vi "Select DB data.vi"(6 "index":i32, 8 "error in (no error)":errorcluster caption="错误输入（无错误）", 9 "Code":string, 10 "Tabe":string, 11 "Connncet State":T1) -> (0 "error out":errorcluster caption="错误输出", 1 "data":string[][](array[string]), 2 "state":bool, 3 "Connect State":T1, 4 "data var":variant[][](array[variant]))   [LabVIEW 2014]
uses:
  <vilib>/addons/database/_DB Variant To Data/Database Variant To Data.xnode
  Ctr/Constr.ctl
  <vilib>/addons/database/Connection.llb/Conn ObjectReference.ctl
  <vilib>/addons/database/NI_Database_API.lvlib
  Ctr/Conneect State.ctl
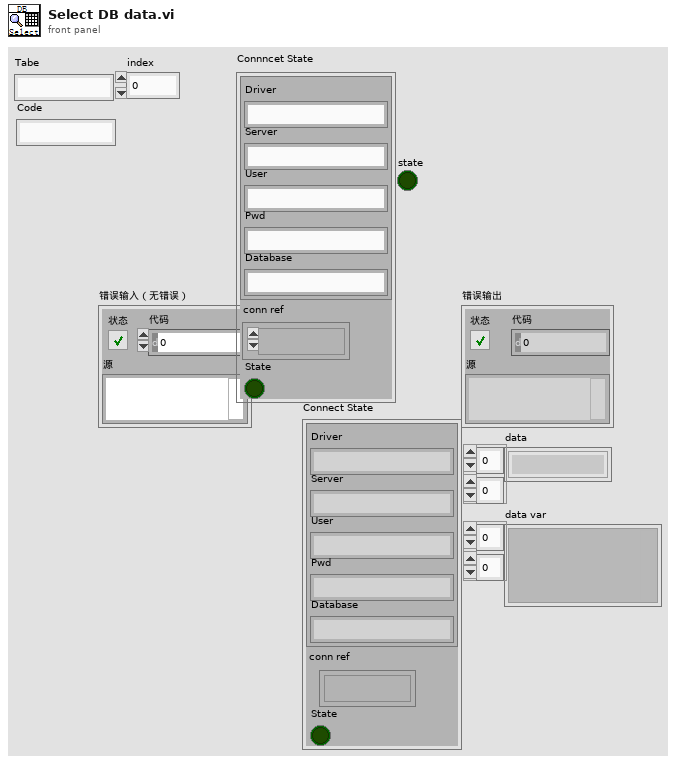
[diagram p1: front panel]
types:
  T1 = typedef "Conneect State.ctl" = cluster{"Constr":T2, "conn ref":T3, "State":bool}
  T2 = typedef "Constr.ctl" = cluster{"Driver":string, "Server":string, "User":string, "Pwd":string, "Database":string}
  T3 = typedef "NI_Database_API.lvlib/Conn ObjectReference.ctl" = refnum<k1>
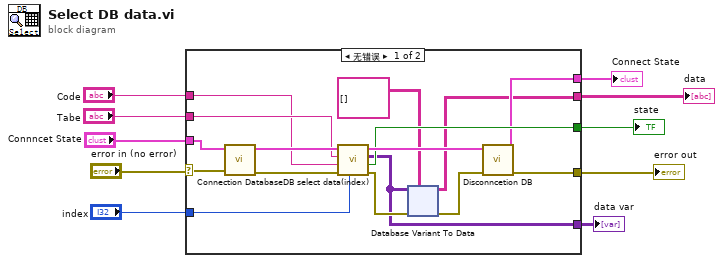
[diagram p0: block diagram]
diagram:
  n1 = case shown="无错误" "error in (no error)" {
    selector: "error in (no error)" -> [w26 w72]
    tunnel: "Connncet State" -> [w25 w71]
    tunnel: [w21 w72] -> w8
    tunnel: "Tabe" -> [w20 _]
    tunnel: "Code" -> [w19 _]
    tunnel: "index" -> [w18 _]
    tunnel: [w17 _] -> w4
    tunnel: [w16 w71] -> w3
    tunnel: [w12 _] -> w2
    tunnel: [w11 _] -> w1
    frame No Error {
      n2 = call "Connection Database.vi"("error in (no error)"=w26, "Connncet State"=w25) -> ("error out"=w24:errorcluster, "Connncet State out"=w23:T1)  [unwired: 8 in]
      n3 = call "DB select data(index).vi"("index"=w18, "error in (no error)"=w24, "Code"=w19, "Tabe"=w20, "Connncet State"=w23) -> ("error out"=w15:errorcluster, "state"=w17:bool, "data"=w11:variant[][], "Connncet State out"=w22:T1)  [unwired: 3 in]
      n4 = xnode "Database Variant To Data"("database variant"=w11, "error in (no error)"=w15, "type"=string[][] []) -> ("data"=w12:string[][], "error out"=w14:errorcluster)
      n5 = call "Disconncetion DB.vi"("error in (no error)"=w14, "Connncet State"=w22) -> ("error out"=w21:errorcluster, "Connect State"=w16:T1)  [unwired: 8 in]
    }
    frame Error {
    }
  }
  "error out" <- w8
  "state" <- w4
  "Connect State" <- w3
  "data" <- w2
  "data var" <- w1
